vi "User_Add.vi"() -> ()   [LabVIEW 2015]
doc: "用于添加，删除新用户，注意权限"
uses:
  <vilib>/registry/registry.llb/Registry RtKey.ctl
  <vilib>/registry/registry.llb/Write Registry Value Simple STR.vi
panel:
  in  "退出":bool caption="取消"
  in  "All User":i32(listbox)
  in  "删除":bool caption="取消"
  in  "添加":bool caption="取消"
  in  "确认密码:":string
  in  "权限":enum16{"学生", "老师"}(ring)
  in  "密码:":string
  in  "新用户名":string
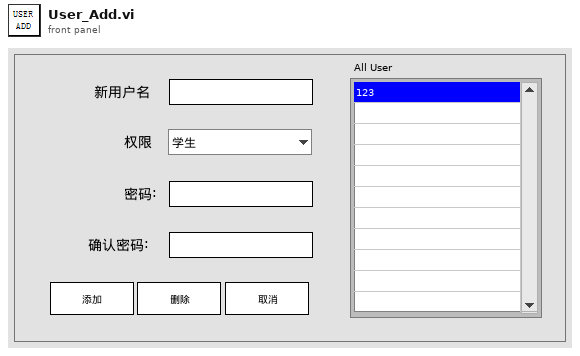
[diagram p1: front panel]
types:
  T1 = typedef "Registry RtKey.ctl" = enum32{"HKEY_CLASSES_ROOT", "HKEY_CURRENT_USER", "HKEY_LOCAL_MACHINE", "HKEY_USERS", "HKEY_PERFORMANCE_DATA", "HKEY_CURRENT_CONFIG", "HKEY_DYN_DATA"}
  T2 = typedef "Registry refnum.ctl" = refnum<k1>
  T3 = cluster{"numValues":i32, "maxValueNameLen":i32, "maxValueDataLen":i32}
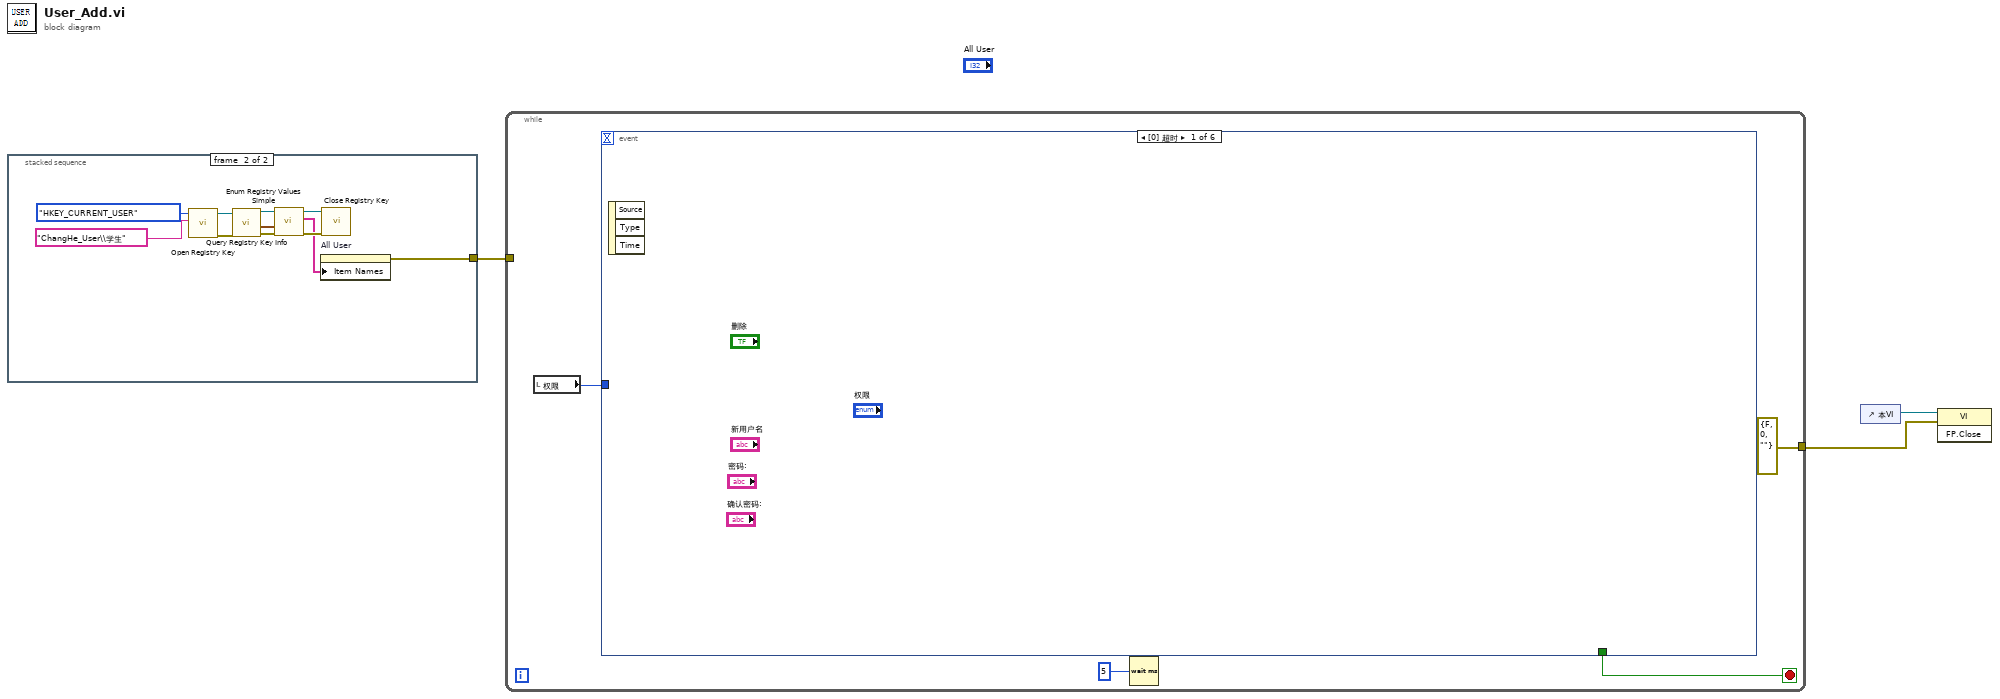
[diagram p0: block diagram]
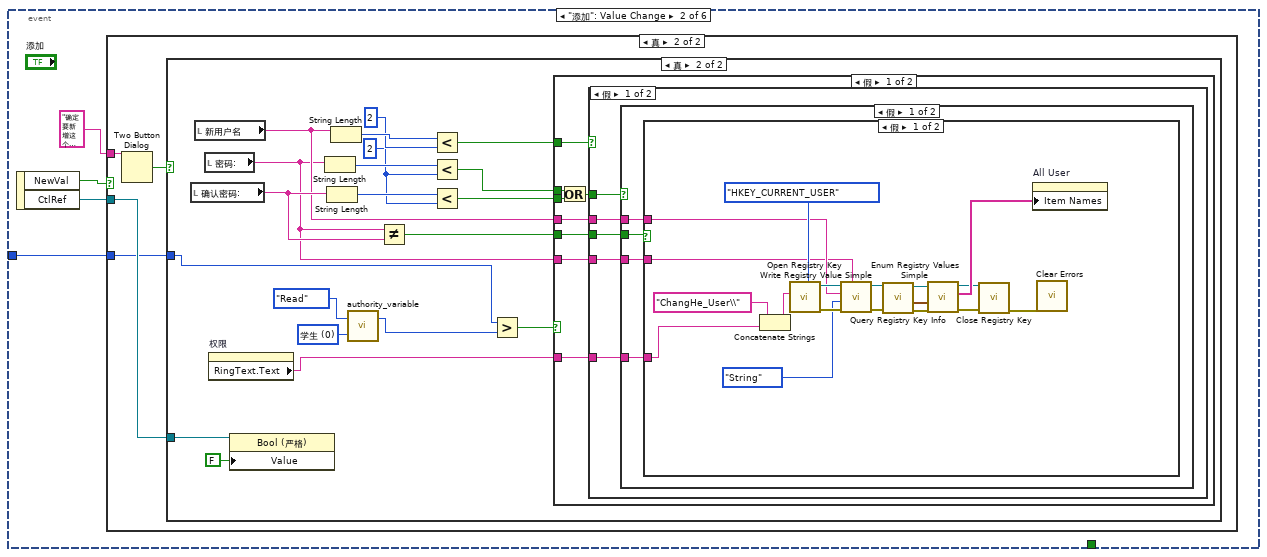
[diagram p2: hidden frame]
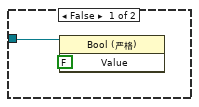
[diagram p4: hidden frame]
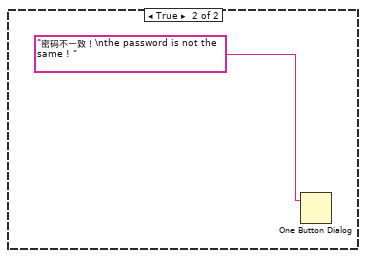
[diagram p5: hidden frame]
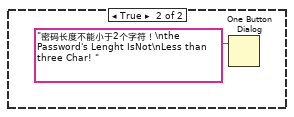
[diagram p6: hidden frame]
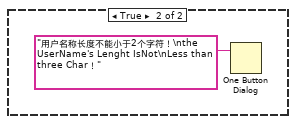
[diagram p7: hidden frame]
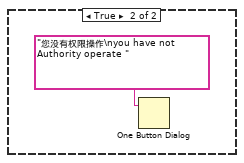
[diagram p8: hidden frame]
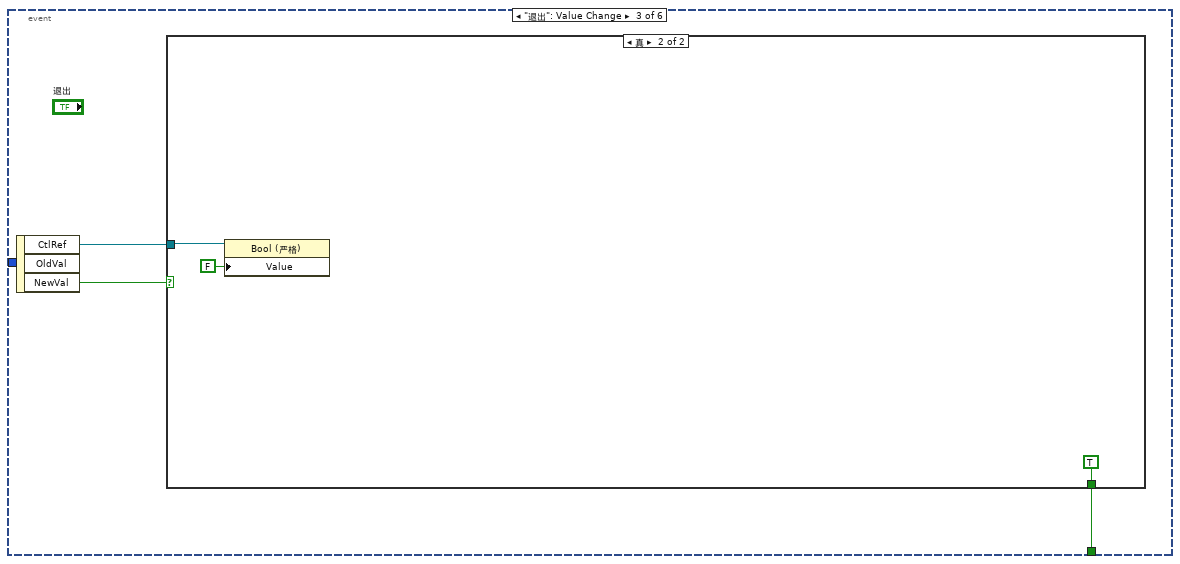
[diagram p9: hidden frame]
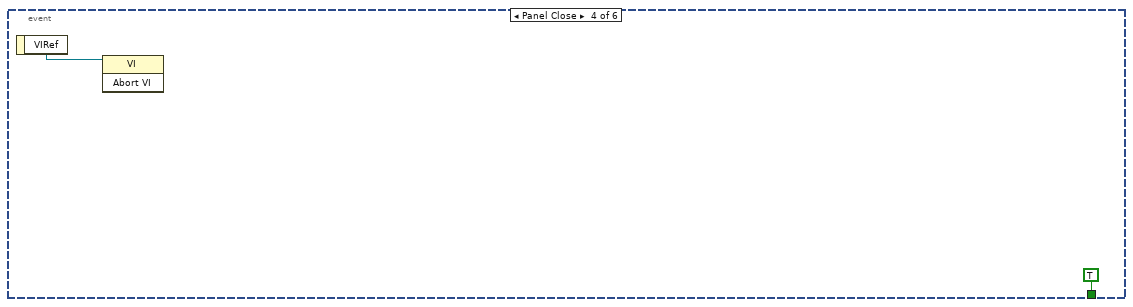
[diagram p11: hidden frame]
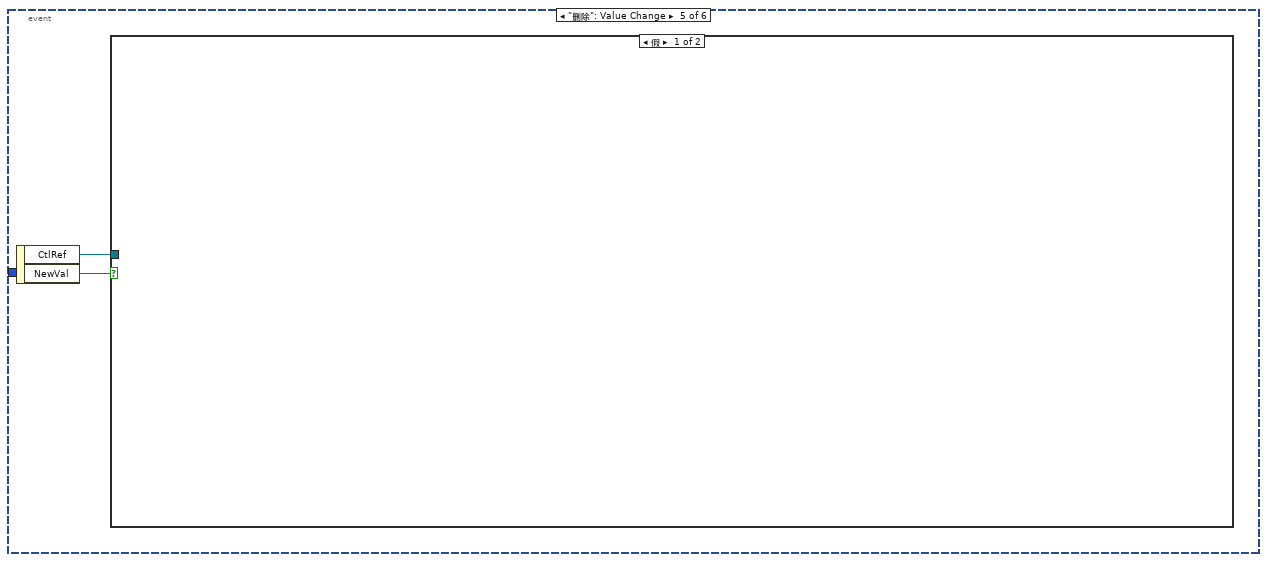
[diagram p12: hidden frame]
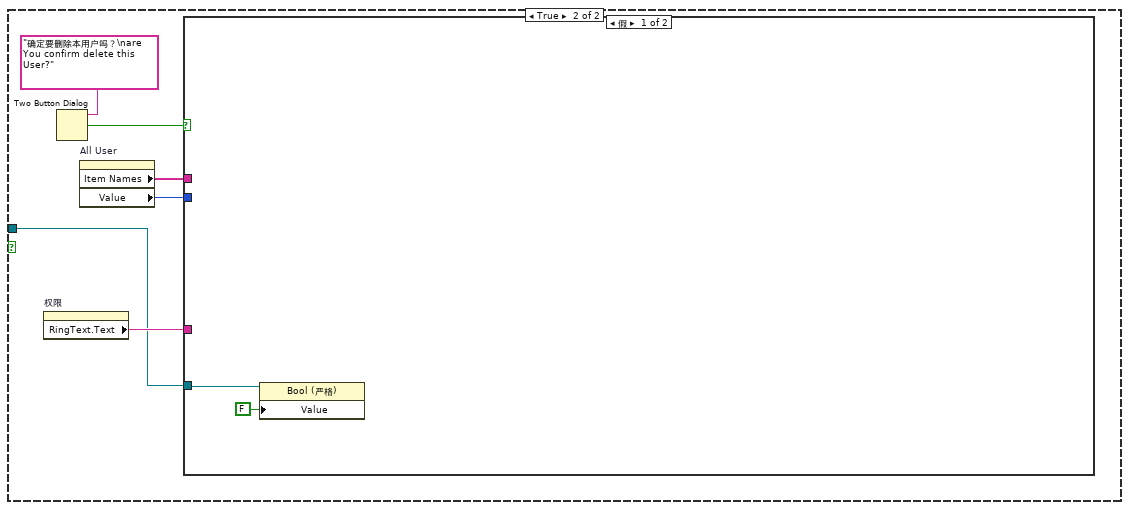
[diagram p13: hidden frame]
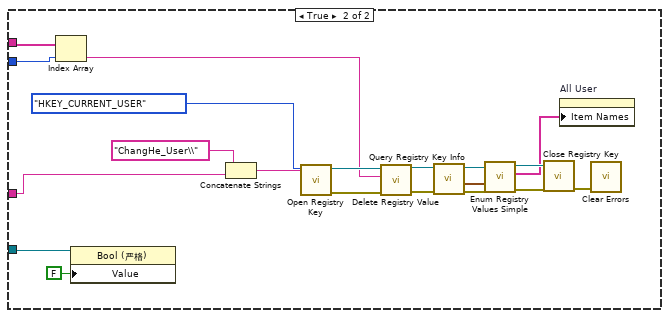
[diagram p14: hidden frame]
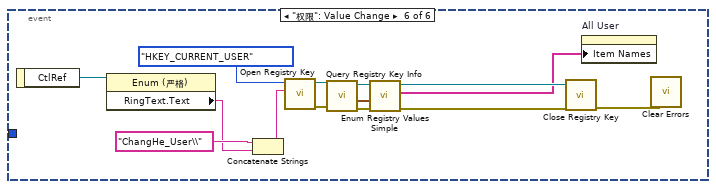
[diagram p15: hidden frame]
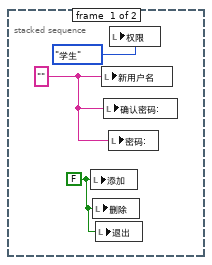
[diagram p16: hidden frame]
diagram:
  n1 = stacked-sequence {
    tunnel: [_ w7] -> w2
    frame #0 {
      w5 = FALSE ("添加")
      w6 = "" ("UserName:")
      n2 = local write "添加"(w5) -> ()
      n3 = local write "删除"(w5) -> ()
      n4 = local write "退出"(w5) -> ()
      n5 = local write "新用户名"(w6) -> ()
      n6 = local write "确认密码:"(w6) -> ()
      n7 = local write "密码:"(w6) -> ()
      n8 = local write "权限"(enum16{"学生", "老师"}."学生" ("权限")) -> ()
    }
    frame #1 {
      n9 = call <vilib>:"Open Registry Key.vi"("subkey"="ChangHe_User\\学生", "root key (HKEY_LOCAL_MACHINE)"=Registry_RtKey."HKEY_CURRENT_USER") -> ("error out"=w15:errorcluster, "refnum out"=w14:T2)  [unwired: 8 in]
      n10 = call <vilib>:"Query Registry Key Info.vi"("error in (no error)"=w15, "refnum"=w14) -> ("error out"=w11:errorcluster, "value info"=w12:T3, "refnum out"=w13:T2)  [unwired: 5 in, 2 out]
      n11 = call <vilib>:"Enum Registry Values Simple.vi"("error in (no error)"=w11, "value info"=w12, "refnum"=w13) -> ("error out"=w10:errorcluster, "values"=w8:string[], "refnum out"=w9:T2)  [unwired: 3 in, 3 out]
      n12 = property on="All User" class="LstBox (严格)"("Item Names"=w8) -> (error out=w7:errorcluster)  [unwired: 2 in, 1 out]
      n13 = call <vilib>:"Close Registry Key.vi"("error in (no error)"=w10, "refnum"=w9) -> ()  [unwired: 5 in, 1 out]
    }
  }
  n14 = while {
    tunnel: [errorcluster {"status"=FALSE, "code"=0, "source"=""} ("错误输入（无错误）")] -> w3
    tunnel: w2 -> [_]
    stop <- w19 stop-if-true
    n15 = local read "权限"() -> (w20:enum16{"学生", "老师"})
    n16 = event shown="[0] 超时" {
      selector: _ -> [_ _ _ _ _ _]
      dyn-events: _ -> [_ _ _ _ _ _]
      timeout: _ -> [_ _ _ _ _ _]
      tunnel: w20 -> [_ w22 _ _ _ _]
      tunnel: [_ _ w91 TRUE _ _] -> w19
      event Timeout {
        n17 = event-data() -> ()  [unwired: 1 in, 3 out]
      }
      event "添加": Value Change {
        n18 = event-data() -> ("NewVal"=w25:bool, "CtlRef"=w23:refnum<vi>)  [unwired: 1 in]
        n19 = case shown="真" w25 {
          tunnel: "确定要新增这个用户吗？\nAre you confirm Add this User ? " ("消息") -> [_ w29]
          tunnel: w23 -> [_ w27]
          tunnel: w22 -> [_ w26]
          frame False {
          }
          frame True {
            n20 = Two Button Dialog(message=w29) -> (T button?=w28:bool)  [unwired: 2 in]
            n21 = case shown="真" w28 {
              tunnel: w27 -> [w30 w38]
              tunnel: w26 -> [_ w34]
              frame False {
                n22 = property class="Bool (严格)"(reference=w30, "Value"=FALSE ("值")) -> ()  [unwired: 1 in, 2 out]
              }
              frame True {
                w32 = u16 0 items=["学生", "老师"] ("Authority_In")
                w47 = 2 ("y")
                n23 = local read "确认密码:"() -> (w41:string)
                n24 = local read "新用户名"() -> (w40:string)
                n25 = local read "密码:"() -> (w39:string)
                n26 = property on="权限" class="Enum (严格)"() -> ("RingText.Text"=w42:string)  [unwired: 2 in, 2 out]
                n27 = property class="Bool (严格)"(reference=w38, "Value"=FALSE ("值")) -> ()  [unwired: 1 in, 2 out]
                n28 = String Length(string=w39) -> (length=w49:i32)
                n29 = String Length(string=w41) -> (length=w48:i32)
                n30 = String Length(string=w40) -> (length=w51:i32)
                n31 = call "authority_variable.vi"("Authority_In"=w32, "select"=enum16{"Read", "Write"}."Read") -> ("Authority_Out"=w33:u16)  [unwired: 1 in]
                n32 = Not Equal?(x=w39, y=w41) -> (x != y?=w43:bool)
                n33 = Less?(x=w51, y=2) -> (x < y?=w46:bool)
                n34 = Less?(x=w49, y=w47) -> (x < y?=w45:bool)
                n35 = Less?(x=w48, y=w47) -> (x < y?=w44:bool)
                n36 = Greater?(x=w34, y=w33) -> (0:w36:bool)
                n37 = case shown="假" w36 {
                  tunnel: w46 -> [w59 _]
                  tunnel: w45 -> [w58 _]
                  tunnel: w44 -> [w57 _]
                  tunnel: w43 -> [w55 _]
                  tunnel: w42 -> [w54 _]
                  tunnel: w40 -> [w53 _]
                  tunnel: w39 -> [w52 _]
                  frame False {
                    n38 = Or(x=w58, y=w57) -> (x .or. y?=w56:bool)
                    n39 = case shown="假" w59 {
                      tunnel: w56 -> [w64 _]
                      tunnel: w55 -> [w63 _]
                      tunnel: w54 -> [w62 _]
                      tunnel: w53 -> [w61 _]
                      tunnel: w52 -> [w60 _]
                      frame False {
                        n40 = case shown="假" w64 {
                          tunnel: w63 -> [w68 _]
                          tunnel: w62 -> [w67 _]
                          tunnel: w61 -> [w66 _]
                          tunnel: w60 -> [w65 _]
                          frame False {
                            n41 = case shown="假" w68 {
                              tunnel: w67 -> [w84 _]
                              tunnel: w66 -> [w80 _]
                              tunnel: w65 -> [w79 _]
                              frame False {
                                n42 = Concatenate Strings("ChangHe_User\\" ("subkey"), w84) -> (w83:string)
                                n43 = call <vilib>:"Open Registry Key.vi"("subkey"=w83, "root key (HKEY_LOCAL_MACHINE)"=Registry_RtKey."HKEY_CURRENT_USER") -> ("error out"=w82:errorcluster, "refnum out"=w81:T2)  [unwired: 8 in]
                                n44 = call-poly <vilib>:"Write Registry Value Simple.vi"("String/Binary data"=w79, "error in (no error)"=w82, "simple data type"=enum16{"String", "Binary", "DWORD"}."String", "value"=w80, "refnum"=w81) -> ("error out"=w78:errorcluster, "refnum out"=w77:T2)  [unwired: 3 in]
                                n45 = call <vilib>:"Query Registry Key Info.vi"("error in (no error)"=w78, "refnum"=w77) -> ("error out"=w76:errorcluster, "value info"=w75:T3, "refnum out"=w74:T2)  [unwired: 5 in, 2 out]
                                n46 = call <vilib>:"Enum Registry Values Simple.vi"("error in (no error)"=w76, "value info"=w75, "refnum"=w74) -> ("error out"=w71:errorcluster, "values"=w73:string[], "refnum out"=w70:T2)  [unwired: 3 in, 3 out]
                                n47 = call <vilib>:"Close Registry Key.vi"("error in (no error)"=w71, "refnum"=w70) -> ("error out"=w69:errorcluster)  [unwired: 5 in]
                                n48 = property on="All User" class="LstBox (严格)"("Item Names"=w73) -> ()  [unwired: 2 in, 2 out]
                                n49 = call <vilib>:"Clear Errors.vi"("error in (no error)"=w69) -> ()  [unwired: 5 in, 2 out]
                              }
                              frame True {
                                n50 = One Button Dialog(message="密码不一致！\nthe password is not the same ! " ("消息")) -> ()  [unwired: 1 in, 1 out]
                              }
                            }
                          }
                          frame True {
                            n51 = One Button Dialog(message="密码长度不能小于2个字符！\nthe Password's Lenght IsNot\nLess than three Char! " ("消息")) -> ()  [unwired: 1 in, 1 out]
                          }
                        }
                      }
                      frame True {
                        n52 = One Button Dialog(message="用户名称长度不能小于2个字符！\nthe UserName's Lenght IsNot\nLess than three Char！" ("消息")) -> ()  [unwired: 1 in, 1 out]
                      }
                    }
                  }
                  frame True {
                    n53 = One Button Dialog(message="您没有权限操作\nyou have not Authority operate " ("消息")) -> ()  [unwired: 1 in, 1 out]
                  }
                }
              }
            }
          }
        }
      }
      event "退出": Value Change {
        n54 = event-data() -> ("CtlRef"=w92:refnum<vi>, "NewVal"=w93:bool)  [unwired: 1 in, 1 out]
        n55 = case shown="真" w93 {
          tunnel: w92 -> [_ w96]
          tunnel: [_ TRUE] -> w91
          frame False {
          }
          frame True {
            n56 = property class="Bool (严格)"(reference=w96, "Value"=FALSE ("值")) -> ()  [unwired: 1 in, 2 out]
          }
        }
      }
      event Panel Close {
        n57 = event-data() -> ("VIRef"=w98:refnum<vi>)  [unwired: 1 in]
        n58 = invoke class="VI" method="Abort VI"(reference=w98) -> ()  [unwired: 2 in, 3 out]
      }
      event "删除": Value Change {
        n59 = event-data() -> ("CtlRef"=w99:refnum<vi>, "NewVal"=w100:bool)  [unwired: 1 in]
        n60 = case shown="假" w100 {
          tunnel: w99 -> [_ w101]
          frame False {
          }
          frame True {
            n61 = property on="权限" class="Enum (严格)"() -> ("RingText.Text"=w104:string)  [unwired: 2 in, 2 out]
            n62 = Two Button Dialog(message="确定要删除本用户吗？\nare You confirm delete this User?" ("消息")) -> (T button?=w105:bool)  [unwired: 2 in]
            n63 = property on="All User" class="LstBox (严格)"() -> ("Item Names"=w103:string[], "Value"=w102:i32)  [unwired: 2 in, 2 out]
            n64 = case shown="假" w105 {
              tunnel: w104 -> [_ w127]
              tunnel: w103 -> [_ w122]
              tunnel: w102 -> [_ w121]
              tunnel: w101 -> [w107 w111]
              frame False {
                n65 = property class="Bool (严格)"(reference=w107, "Value"=FALSE ("值")) -> ()  [unwired: 1 in, 2 out]
              }
              frame True {
                n66 = Index Array(array=w122, index=w121) -> (element=w120:string)
                n67 = property class="Bool (严格)"(reference=w111, "Value"=FALSE ("值")) -> ()  [unwired: 1 in, 2 out]
                n68 = Concatenate Strings("ChangHe_User\\" ("subkey"), w127) -> (w126:string)
                n69 = call <vilib>:"Open Registry Key.vi"("subkey"=w126, "root key (HKEY_LOCAL_MACHINE)"=Registry_RtKey."HKEY_CURRENT_USER") -> ("error out"=w123:errorcluster, "refnum out"=w124:T2)  [unwired: 8 in]
                n70 = call <vilib>:"Delete Registry Value.vi"("error in (no error)"=w123, "value"=w120, "refnum"=w124) -> ("error out"=w118:errorcluster, "refnum out"=w119:T2)  [unwired: 7 in]
                n71 = call <vilib>:"Query Registry Key Info.vi"("error in (no error)"=w118, "refnum"=w119) -> ("error out"=w117:errorcluster, "value info"=w116:T3, "refnum out"=w115:T2)  [unwired: 5 in, 2 out]
                n72 = call <vilib>:"Enum Registry Values Simple.vi"("error in (no error)"=w117, "value info"=w116, "refnum"=w115) -> ("error out"=w114:errorcluster, "values"=w112:string[], "refnum out"=w113:T2)  [unwired: 3 in, 3 out]
                n73 = call <vilib>:"Close Registry Key.vi"("error in (no error)"=w114, "refnum"=w113) -> ("error out"=w109:errorcluster)  [unwired: 5 in]
                n74 = property on="All User" class="LstBox (严格)"("Item Names"=w112) -> ()  [unwired: 2 in, 2 out]
                n75 = call <vilib>:"Clear Errors.vi"("error in (no error)"=w109) -> ()  [unwired: 5 in, 2 out]
              }
            }
          }
        }
      }
      event "权限": Value Change {
        n76 = event-data() -> ("CtlRef"=w142:refnum<vi>)  [unwired: 1 in]
        n77 = property class="Enum (严格)"(reference=w142) -> ("RingText.Text"=w139:string)  [unwired: 1 in, 2 out]
        n78 = Concatenate Strings("ChangHe_User\\" ("subkey"), w139) -> (w140:string)
        n79 = call <vilib>:"Open Registry Key.vi"("subkey"=w140, "root key (HKEY_LOCAL_MACHINE)"=Registry_RtKey."HKEY_CURRENT_USER") -> ("error out"=w137:errorcluster, "refnum out"=w136:T2)  [unwired: 8 in]
        n80 = call <vilib>:"Query Registry Key Info.vi"("error in (no error)"=w137, "refnum"=w136) -> ("error out"=w135:errorcluster, "value info"=w134:T3, "refnum out"=w133:T2)  [unwired: 5 in, 2 out]
        n81 = call <vilib>:"Enum Registry Values Simple.vi"("error in (no error)"=w135, "value info"=w134, "refnum"=w133) -> ("error out"=w132:errorcluster, "values"=w130:string[], "refnum out"=w131:T2)  [unwired: 3 in, 3 out]
        n82 = call <vilib>:"Close Registry Key.vi"("error in (no error)"=w132, "refnum"=w131) -> ("error out"=w129:errorcluster)  [unwired: 5 in]
        n83 = property on="All User" class="LstBox (严格)"("Item Names"=w130) -> ()  [unwired: 2 in, 2 out]
        n84 = call <vilib>:"Clear Errors.vi"("error in (no error)"=w129) -> ()  [unwired: 5 in, 2 out]
      }
    }
    n85 = Wait (ms)(milliseconds to wait=u32 5 ("等待时间（毫秒）")) -> ()  [unwired: 1 out]
  }
  n86 = control-ref of="本VI"() -> (w1:refnum<vi>)
  n87 = invoke class="VI" method="FP.Close"(reference=w1, error in=w3) -> ()  [unwired: 1 in, 3 out]
